vi "UHR-Fleezers Control (host) - 11.9.vi"() -> ()   [LabVIEW 2014] (continued)
                                n672 = Select(t=w978, s="Random Choice", f=w984) -> (s? t:f=w982:dbl)
                                n673 = Select(t="Yank to Trap D (MHz)", s="Yank to which?", f="Yank to SP") -> (s? t:f=w975:dbl[])
                                n674 = Index Array(array=w975, index=w982) -> (element=w985:dbl)
                                n675 = case shown="False" "Yank to which?" {
                                tunnel: w985 -> [w986 w1013]
                                frame False {
                                n676 = flat-sequence {
                                tunnel: w986 -> [w987]
                                frame #0 {
                                n677 = property on="Trap Pos FB SP" class="DigNum (strict)"("Val(Sgnl)"=w987) -> ()  [unwired: 2 in, 2 out]
                                }
                                frame #1 {
                                n678 = Wait (ms)(milliseconds to wait=u32 700) -> ()  [unwired: 1 out]
                                }
                                frame #2 {
                                n679 = local read "Action (%)"() -> (w992:dbl)
                                n680 = Absolute Value(x=w992) -> (abs(x)=w991:dbl)
                                n681 = Greater?(x=w991, y=70.0) -> (0:w989:bool)
                                n682 = property on="Remove Action Offset" class="Bool (strict)"("Val(Sgnl)"=w989) -> ()  [unwired: 2 in, 2 out]
                                }
                                frame #3 {
                                n683 = for {
                                N: 4 -> [_]
                                n684 = flat-sequence {
                                frame #0 {
                                n685 = Wait (ms)(milliseconds to wait=u32 500) -> ()  [unwired: 1 out]
                                }
                                frame #1 {
                                n686 = local read "Action (%)"() -> (w998:dbl)
                                n687 = Absolute Value(x=w998) -> (abs(x)=w997:dbl)
                                n688 = Greater?(x=w997, y=70.0) -> (0:w995:bool)
                                n689 = property on="Remove Action Offset" class="Bool (strict)"("Val(Sgnl)"=w995) -> ()  [unwired: 2 in, 2 out]
                                }
                                }
                                }
                                }
                                frame #4 {
                                n690 = local read "Shift confocal"() -> (w1002:bool)
                                n691 = local read "Mean"() -> (w1005:dbl)
                                n692 = Greater?(x=w1005, y=11.0) -> (0:w1001:bool)
                                n693 = Not(x=w1001) -> (.not. x?=w1000:bool)
                                n694 = And(x=w1000, y=w1002) -> (x .and. y?=w999:bool)
                                n695 = And(x=w1001, y=w1002) -> (x .and. y?=w1003:bool)
                                n696 = case shown="True" w1003 {
                                frame False {
                                }
                                frame True {
                                n697 = local read "Confocal X 2 (V)"() -> (w1008:dbl)
                                n698 = local read "Confocal Y 2 (V)"() -> (w1009:dbl)
                                n699 = property on="AO2" class="Slide (strict)"("Val(Sgnl)"=w1008) -> ()  [unwired: 2 in, 2 out]
                                n700 = property on="AO1" class="Slide (strict)"("Val(Sgnl)"=w1009) -> ()  [unwired: 2 in, 2 out]
                                }
                                }
                                n701 = case shown="True" w999 {
                                frame False {
                                }
                                frame True {
                                n702 = local read "Confocal X 1 (V)"() -> (w1006:dbl)
                                n703 = local read "Confocal Y 1 (V)"() -> (w1007:dbl)
                                n704 = property on="AO1" class="Slide (strict)"("Val(Sgnl)"=w1007) -> ()  [unwired: 2 in, 2 out]
                                n705 = property on="AO2" class="Slide (strict)"("Val(Sgnl)"=w1006) -> ()  [unwired: 2 in, 2 out]
                                }
                                }
                                }
                                frame #5 {
                                n706 = Wait (ms)(milliseconds to wait=u32 1500) -> ()  [unwired: 1 out]
                                }
                                frame #6 {
                                n707 = property on="Remove Offset" class="Bool (strict)"("Val(Sgnl)"=TRUE ("Value (Signaling)")) -> ()  [unwired: 2 in, 2 out]
                                n708 = property on="Rem fb disp offset" class="Bool (strict)"("Val(Sgnl)"=TRUE ("Value (Signaling)")) -> ()  [unwired: 2 in, 2 out]
                                }
                                }
                                }
                                frame True {
                                n709 = flat-sequence {
                                tunnel: w1013 -> [w1014]
                                frame #0 {
                                n710 = property on="Trap D (MHz)" class="DigNum (strict)"("Val(Sgnl)"=w1014) -> ()  [unwired: 2 in, 2 out]
                                }
                                frame #1 {
                                n711 = Wait (ms)(milliseconds to wait=u32 500) -> ()  [unwired: 1 out]
                                }
                                frame #2 {
                                n712 = local read "Shift confocal"() -> (w1018:bool)
                                n713 = local read "Mean"() -> (w1016:dbl)
                                n714 = Greater?(x=w1016, y=11.0) -> (0:w1019:bool)
                                n715 = Not(x=w1019) -> (.not. x?=w1020:bool)
                                n716 = And(x=w1020, y=w1018) -> (x .and. y?=w1022:bool)
                                n717 = And(x=w1019, y=w1018) -> (x .and. y?=w1021:bool)
                                n718 = case shown="True" w1021 {
                                frame False {
                                }
                                frame True {
                                n719 = local read "Confocal Y 2 (V)"() -> (w1026:dbl)
                                n720 = local read "Confocal X 2 (V)"() -> (w1025:dbl)
                                n721 = property on="AO1" class="Slide (strict)"("Val(Sgnl)"=w1026) -> ()  [unwired: 2 in, 2 out]
                                n722 = property on="AO2" class="Slide (strict)"("Val(Sgnl)"=w1025) -> ()  [unwired: 2 in, 2 out]
                                }
                                }
                                n723 = case shown="True" w1022 {
                                frame False {
                                }
                                frame True {
                                n724 = local read "Confocal X 1 (V)"() -> (w1023:dbl)
                                n725 = local read "Confocal Y 1 (V)"() -> (w1024:dbl)
                                n726 = property on="AO2" class="Slide (strict)"("Val(Sgnl)"=w1023) -> ()  [unwired: 2 in, 2 out]
                                n727 = property on="AO1" class="Slide (strict)"("Val(Sgnl)"=w1024) -> ()  [unwired: 2 in, 2 out]
                                }
                                }
                                }
                                }
                                }
                                }
                                }
                              }
                            }
                            frame "Raster" {
                              n728 = property on="Trap Raster Scan" class="Bool (strict)"("Val(Sgnl)"=TRUE ("Value (Signaling)")) -> ()  [unwired: 2 in, 2 out]
                            }
                          }
                          n729 = local read "Time (s)"() -> (w959:dbl)
                          "Fl. High" <- TRUE ("Yanking")
                        }
                        frame #1 {
                          n730 = local read "Auto F Reset"() -> (w1028:bool)
                          n731 = case shown="True" w1028 {
                            tunnel: w1033 -> [_ w1037]
                            tunnel: w1032 -> [_ w1036]
                            tunnel: w1031 -> [_ w1035]
                            tunnel: w1029 -> [_ w1034]
                            frame False {
                            }
                            frame True {
                              n732 = node-c288() -> (w1039:T21)  [unwired: 4 out]
                              n733 = timed-loop {
                                timing: w1039 -> [_]
                                timing-out: [_] -> w1038
                                tunnel: w1037 -> [w1057]
                                tunnel: w1036 -> [w1056]
                                tunnel: w1035 -> [w1055]
                                tunnel: w1034 -> [w1054]
                                stop <- w1040 stop-if-true
                                n734 = node-c288() -> ()  [unwired: 2 out]
                                n735 = local read "Fl. D Thresh. (kHz)"() -> (w1048:dbl)
                                n736 = local read "Fl. Triggered..."() -> (w1053:bool)
                                n737 = local read "Delta Fl. 1"() -> (w1044:dbl)
                                n738 = local read "Delta Fl. 2"() -> (w1042:dbl)
                                n739 = local read "Stop All"() -> (w1051:bool)
                                n740 = local read "APD to Watch"() -> (w1043:bool)
                                n741 = Select(t=w1044, s=w1043, f=w1042) -> (s? t:f=w1041:dbl)
                                n742 = Not(x=w1053) -> (.not. x?=w1052:bool)
                                n743 = Multiply(x=w1048, y=1000.0) -> (x*y=w1047:dbl)
                                n744 = Negate(x=w1047) -> (-x=w1046:dbl)
                                n745 = Less?(x=w1041, y=w1046) -> (x < y?=w1050:bool)
                                n746 = Compound Arithmetic op=OR(w1050, w1051, w1052, "Reset Force") -> (w1040:bool)
                                n747 = case shown="True" w1040 {
                                tunnel: w1057 -> [_ w1072]
                                tunnel: w1056 -> [_ w1071]
                                tunnel: w1055 -> [_ w1061]
                                tunnel: w1054 -> [_ w1063]
                                frame False {
                                }
                                frame True {
                                n748 = local read "Time (s)"() -> (w1062:dbl)
                                n749 = case shown="\"Yank\"" w1071 {
                                tunnel: w1072 -> [_ w1075]
                                tunnel: w1063 -> [_ w1073]
                                frame "Image", Default {
                                }
                                frame "Yank" {
                                n750 = flat-sequence {
                                tunnel: [w1081] -> w1076
                                tunnel: w1075 -> [w1081]
                                tunnel: [w1077] -> w1074
                                tunnel: w1073 -> [w1077]
                                tunnel: w1076 -> [w1084]
                                tunnel: w1074 -> [w1082]
                                frame #0 {
                                n751 = local read "Yank Delay (s)"() -> (w1080:dbl)
                                n752 = Multiply(x=w1080, y=1000.0) -> (x*y=w1078:dbl)
                                n753 = Wait (ms)(milliseconds to wait=w1078) -> ()  [unwired: 1 out]
                                }
                                frame #1 {
                                n754 = local read "Yank to which?"() -> (w1083:bool)
                                n755 = case shown="False" w1083 {
                                tunnel: w1084 -> [_ w1112]
                                tunnel: w1082 -> [w1085 _]
                                frame False {
                                n756 = flat-sequence {
                                tunnel: w1085 -> [w1086]
                                frame #0 {
                                n757 = property on="Trap Pos FB SP" class="DigNum (strict)"("Val(Sgnl)"=w1086) -> ()  [unwired: 2 in, 2 out]
                                }
                                frame #1 {
                                n758 = Wait (ms)(milliseconds to wait=u32 700) -> ()  [unwired: 1 out]
                                }
                                frame #2 {
                                n759 = local read "Action (%)"() -> (w1091:dbl)
                                n760 = Absolute Value(x=w1091) -> (abs(x)=w1090:dbl)
                                n761 = Greater?(x=w1090, y=70.0) -> (0:w1088:bool)
                                n762 = property on="Remove Action Offset" class="Bool (strict)"("Val(Sgnl)"=w1088) -> ()  [unwired: 2 in, 2 out]
                                }
                                frame #3 {
                                n763 = for {
                                N: 4 -> [_]
                                n764 = flat-sequence {
                                frame #0 {
                                n765 = Wait (ms)(milliseconds to wait=u32 500) -> ()  [unwired: 1 out]
                                }
                                frame #1 {
                                n766 = local read "Action (%)"() -> (w1097:dbl)
                                n767 = Absolute Value(x=w1097) -> (abs(x)=w1096:dbl)
                                n768 = Greater?(x=w1096, y=70.0) -> (0:w1094:bool)
                                n769 = property on="Remove Action Offset" class="Bool (strict)"("Val(Sgnl)"=w1094) -> ()  [unwired: 2 in, 2 out]
                                }
                                }
                                }
                                }
                                frame #4 {
                                n770 = local read "Shift confocal"() -> (w1102:bool)
                                n771 = local read "Mean"() -> (w1104:dbl)
                                n772 = Greater?(x=w1104, y=11.0) -> (0:w1101:bool)
                                n773 = Not(x=w1101) -> (.not. x?=w1100:bool)
                                n774 = And(x=w1101, y=w1102) -> (x .and. y?=w1099:bool)
                                n775 = And(x=w1100, y=w1102) -> (x .and. y?=w1098:bool)
                                n776 = case shown="True" w1099 {
                                frame False {
                                }
                                frame True {
                                n777 = local read "Confocal Y 2 (V)"() -> (w1108:dbl)
                                n778 = local read "Confocal X 2 (V)"() -> (w1107:dbl)
                                n779 = property on="AO2" class="Slide (strict)"("Val(Sgnl)"=w1107) -> ()  [unwired: 2 in, 2 out]
                                n780 = property on="AO1" class="Slide (strict)"("Val(Sgnl)"=w1108) -> ()  [unwired: 2 in, 2 out]
                                }
                                }
                                n781 = case shown="True" w1098 {
                                frame False {
                                }
                                frame True {
                                n782 = local read "Confocal X 1 (V)"() -> (w1105:dbl)
                                n783 = local read "Confocal Y 1 (V)"() -> (w1106:dbl)
                                n784 = property on="AO1" class="Slide (strict)"("Val(Sgnl)"=w1106) -> ()  [unwired: 2 in, 2 out]
                                n785 = property on="AO2" class="Slide (strict)"("Val(Sgnl)"=w1105) -> ()  [unwired: 2 in, 2 out]
                                }
                                }
                                }
                                frame #5 {
                                n786 = Wait (ms)(milliseconds to wait=u32 1500) -> ()  [unwired: 1 out]
                                }
                                frame #6 {
                                n787 = property on="Rem fb disp offset" class="Bool (strict)"("Val(Sgnl)"=TRUE ("Value (Signaling)")) -> ()  [unwired: 2 in, 2 out]
                                n788 = property on="Remove Offset" class="Bool (strict)"("Val(Sgnl)"=TRUE ("Value (Signaling)")) -> ()  [unwired: 2 in, 2 out]
                                }
                                }
                                }
                                frame True {
                                n789 = flat-sequence {
                                tunnel: w1112 -> [w1113]
                                frame #0 {
                                n790 = property on="Trap D (MHz)" class="DigNum (strict)"("Val(Sgnl)"=w1113) -> ()  [unwired: 2 in, 2 out]
                                }
                                frame #1 {
                                n791 = Wait (ms)(milliseconds to wait=u32 500) -> ()  [unwired: 1 out]
                                }
                                frame #2 {
                                n792 = local read "Shift confocal"() -> (w1119:bool)
                                n793 = local read "Mean"() -> (w1121:dbl)
                                n794 = Greater?(x=w1121, y=11.0) -> (0:w1118:bool)
                                n795 = Not(x=w1118) -> (.not. x?=w1117:bool)
                                n796 = And(x=w1118, y=w1119) -> (x .and. y?=w1116:bool)
                                n797 = And(x=w1117, y=w1119) -> (x .and. y?=w1115:bool)
                                n798 = case shown="True" w1116 {
                                frame False {
                                }
                                frame True {
                                n799 = local read "Confocal Y 2 (V)"() -> (w1125:dbl)
                                n800 = local read "Confocal X 2 (V)"() -> (w1124:dbl)
                                n801 = property on="AO2" class="Slide (strict)"("Val(Sgnl)"=w1124) -> ()  [unwired: 2 in, 2 out]
                                n802 = property on="AO1" class="Slide (strict)"("Val(Sgnl)"=w1125) -> ()  [unwired: 2 in, 2 out]
                                }
                                }
                                n803 = case shown="True" w1115 {
                                frame False {
                                }
                                frame True {
                                n804 = local read "Confocal Y 1 (V)"() -> (w1123:dbl)
                                n805 = local read "Confocal X 1 (V)"() -> (w1122:dbl)
                                n806 = property on="AO2" class="Slide (strict)"("Val(Sgnl)"=w1122) -> ()  [unwired: 2 in, 2 out]
                                n807 = property on="AO1" class="Slide (strict)"("Val(Sgnl)"=w1123) -> ()  [unwired: 2 in, 2 out]
                                }
                                }
                                }
                                }
                                }
                                }
                                }
                                }
                                }
                                }
                                n808 = local read "Messages"() -> (w1070:string)
                                n809 = Subtract(x=w1062, y=w1061) -> (x-y=w1068:dbl)
                                "Duration (s)" <- w1068
                                n810 = Number To Decimal String(number=w1068, width (-)=i16 0) -> (decimal integer string=w1066:string)
                                n811 = Concatenate Strings(w1066, " s fluorescence event." ("string")) -> (w1064:string)
                                n812 = call "Update messages.vi"("Message to add"=w1064, "Old message string"=w1070) -> ("New message string"=w1069:string)
                                n813 = local write "Reset Force"(FALSE ("Reset Force")) -> ()
                                n814 = local write "Waiting"(TRUE ("Waiting")) -> ()
                                n815 = local write "Messages"(w1069) -> ()
                                n816 = local write "Fl. High"(FALSE ("Fl. High")) -> ()
                                n817 = call <vilib>:"Beep.vi"() -> ()  [unwired: 3 in, 9 out]
                                }
                                }
                                n818 = node-c288() -> ()  [unwired: 2 out]
                              }
                              n819 = node-c288(w1038) -> ()  [unwired: 1 out]
                            }
                          }
                        }
                      }
                      n820 = local read "Trap Pos FB SP"() -> (w946:fxp<+/-,16,1>)
                      n821 = local read "Trap D (MHz)"() -> (w951:dbl)
                    }
                  }
                }
                frame #1 {
                  n822 = local read "Stop All"() -> (w1135:bool)
                  n823 = local read "Fl. Triggered..."() -> (w1133:bool)
                  n824 = Not(x=w1133) -> (.not. x?=w1134:bool)
                  n825 = Or(x=w1134, y=w1135) -> (x .or. y?=w1132:bool)
                }
              }
              n826 = case shown="True" w721 {
                frame False {
                }
                frame True {
                  n827 = local read "Confocal Y 1 (V)"() -> (w731:dbl)
                  n828 = local read "Confocal X 1 (V)"() -> (w730:dbl)
                  n829 = property on="AO2" class="Slide (strict)"("Val(Sgnl)"=w730) -> ()  [unwired: 2 in, 2 out]
                  n830 = property on="AO1" class="Slide (strict)"("Val(Sgnl)"=w731) -> ()  [unwired: 2 in, 2 out]
                }
              }
              n831 = case shown="True" w721 {
                frame False {
                }
                frame True {
                  w729 = FALSE ("Fl. High")
                  n832 = local write "Waiting"(w729) -> ()
                  n833 = local write "Fl. High"(w729) -> ()
                }
              }
              n834 = node-c288() -> ()  [unwired: 2 out]
            }
            n835 = node-c288(w719) -> ()  [unwired: 1 out]
          }
        }
      }
      event "Stop All": Value Change {
        n836 = event-data() -> ()  [unwired: 7 out]
        n837 = local read "Stop All"() -> (w1140:bool)
      }
    }
    n838 = node-c288() -> ()  [unwired: 2 out]
  }
  n839 = property on="Saved trap pos" class="WFGraph (strict)"("Visible"=TRUE) -> ()  [unwired: 2 in, 2 out]
  n840 = property on="Trap Delta Graph" class="WFGraph (strict)"("Visible"=FALSE) -> ()  [unwired: 2 in, 2 out]
  n841 = local write "Trap pos"(TRUE ("Trap pos")) -> ()
  n842 = node-c288(2 ("Processor")) -> (w110:T21)  [unwired: 3 out]
  n843 = timed-loop "Control parameters (event loop)" {
    tunnel: w20 -> [w1149]
    shift-right: [w1148] -> _
    shift-left: errorcluster {"status"=FALSE, "code"=0, "source"=""} ("error out") -> [w1147]
    tunnel: [w1146] -> _
    timing: w110 -> [_]
    timing-out: [_] -> w109
    tunnel: w83 -> [w1145]
    tunnel: w24 -> [w1144]
    tunnel: w23 -> [w1143]
    tunnel: w22 -> [w1142]
    tunnel: w21 -> [w1141]
    stop <- w1146 stop-if-true
    n844 = node-c288() -> ()  [unwired: 2 out]
    n845 = event shown="[77] \"Save user params\": Value Change" {
      selector: _ -> [_ _ _ _ _ _ _ _ _ _ _ _ _ _ _ _ _ _ _ _ _ _ _ _ _ _ _ _ _ _ _ _ _ _ _ _ _ _ _ _ _ _ _ _ _ _ _ _ _ _ _ _ _ _ _ _ _ _ _ _ _ _ _ _ _ _ _ _ _ _ _ _ _ _ _ _ _ _ _ _]
      dyn-events: _ -> [_ _ _ _ _ _ _ _ _ _ _ _ _ _ _ _ _ _ _ _ _ _ _ _ _ _ _ _ _ _ _ _ _ _ _ _ _ _ _ _ _ _ _ _ _ _ _ _ _ _ _ _ _ _ _ _ _ _ _ _ _ _ _ _ _ _ _ _ _ _ _ _ _ _ _ _ _ _ _ _]
      timeout: _ -> [_ _ _ _ _ _ _ _ _ _ _ _ _ _ _ _ _ _ _ _ _ _ _ _ _ _ _ _ _ _ _ _ _ _ _ _ _ _ _ _ _ _ _ _ _ _ _ _ _ _ _ _ _ _ _ _ _ _ _ _ _ _ _ _ _ _ _ _ _ _ _ _ _ _ _ _ _ _ _ _]
      tunnel: w1149 -> [w1187 _ _ _ w1225 _ w1247 _ _ _ _ w1313 _ _ w1356 w1362 w1367 w1373 w1409 w1427 w1434 _ w1446 w1450 w1461 w1472 w1483 w1494 w1505 w1516 w1543 w1637 w1644 w1682 _ _ w1742 w1746 w1757 w1761 w1765 _ w1773 _ _ _ _ _ _ _ _ _ _ _ _ _ _ _ _ _ w2154 _ w2171 _ w2178 w2196 _ w2203 w2211 w2226 w2237 w2243 _ w2252 _ w2271 _ _ _ w2346]
      tunnel: [w1186 _ _ _ w1215 _ w1246 _ _ w1278 _ w1292 _ _ w1355 w1358 w1364 w1370 w1408 w1425 w1433 _ w1444 _ w1455 w1466 w1477 w1488 w1499 w1510 w1541 w1635 w1642 w1680 _ _ w1740 w1744 w1747 w1759 w1763 _ w1771 _ _ _ _ _ _ _ _ _ _ _ _ _ _ _ _ _ w2152 _ _ _ _ w2193 _ _ _ _ _ _ _ _ _ _ _ _ _ w2344] -> w1148
      tunnel: w1147 -> [w1185 _ _ _ w1224 _ w1245 _ _ w1278 _ w1312 _ _ w1354 w1357 w1363 w1369 w1407 w1426 w1432 _ w1445 w1449 w1460 w1471 w1482 w1493 w1504 w1515 w1542 w1636 w1643 w1681 _ _ w1741 w1745 w1756 w1760 w1764 _ w1772 _ _ _ _ _ _ _ _ _ _ _ _ _ _ _ _ _ w2153 _ w2170 _ w2177 w2195 _ w2202 w2210 w2225 w2236 w2242 _ w2251 _ w2270 _ _ _ w2345]
      tunnel: [_ _ _ _ _ _ _ _ _ w1277 _ _ _ _ _ _ _ _ _ _ _ _ _ _ _ _ _ _ _ _ _ _ _ _ _ _ _ _ _ _ _ _ _ _ _ _ _ _ _ _ _ _ _ _ _ _ _ _ _ _ _ _ _ _ _ _ _ _ _ _ _ _ _ _ _ _ _ _ _ _] -> w1146
      tunnel: [_ _ _ _ _ _ _ "Round T1 X" _ _ _ _ _ _ _ _ _ _ _ _ _ _ _ _ _ _ _ _ _ _ _ _ _ _ _ _ _ _ _ _ _ _ _ _ _ _ _ _ _ _ _ _ _ _ _ _ _ _ _ _ _ _ _ _ _ _ _ _ _ _ _ _ _ _ _ _ _ _ _ _] -> _
      tunnel: [_ _ _ "Adjust Scale\nto Mean" _ _ _ _ _ _ _ _ _ _ _ _ _ _ _ _ _ _ "Test ttrig" _ _ _ _ _ _ _ _ _ _ _ _ _ _ _ _ _ _ _ _ _ _ _ _ _ _ _ "Flush Sample" "Flush Pump 3" "Flush Pump 1" "Clear Volume" _ _ _ _ _ _ _ _ _ _ _ _ _ _ _ _ _ _ _ _ _ _ _ _ _ _] -> _
      tunnel: [_ _ _ _ _ _ _ _ "Round T2 X" _ "Delayed Interlace Start" _ _ _ _ _ _ _ _ _ _ _ _ _ _ _ _ _ _ _ _ _ _ _ _ _ _ _ _ _ _ _ _ _ _ _ _ _ _ _ _ _ _ _ _ _ _ _ _ _ _ _ _ _ _ _ _ _ _ _ _ _ _ _ _ _ _ _ _ _] -> _
      tunnel: w1145 -> [_ _ _ _ _ _ _ _ _ _ _ _ _ _ _ _ _ _ _ _ _ _ _ _ _ _ _ _ _ _ _ _ _ _ _ _ _ _ _ _ _ _ _ _ _ _ w1931 w1949 w1956 w1961 w1967 _ _ w2066 _ _ _ _ _ _ _ _ _ _ _ _ _ _ _ _ _ _ _ _ _ _ _ _ _ _]
      tunnel: w1144 -> [_ _ _ _ _ _ _ _ _ _ _ _ _ _ _ _ _ _ _ _ _ _ _ _ _ _ _ _ _ _ _ _ _ _ _ _ _ _ _ _ _ _ _ _ w1847 _ _ _ _ _ _ w1997 _ _ w2073 _ w2082 _ w2096 _ _ _ _ _ _ _ _ _ _ _ _ _ _ _ _ _ _ _ _ _]
      tunnel: w1143 -> [_ _ _ _ _ _ _ _ _ _ _ _ _ _ _ _ _ _ _ _ _ _ _ _ _ _ _ _ _ _ _ _ _ _ _ _ _ _ _ _ _ _ _ _ _ _ _ _ _ _ _ _ _ _ _ _ _ _ _ _ _ _ _ _ _ _ _ _ _ _ _ _ _ _ _ _ _ _ _ _]
      tunnel: w1142 -> [_ _ _ _ _ _ _ _ _ _ _ _ _ _ _ _ _ _ _ _ _ _ _ _ _ _ _ _ _ _ _ _ _ _ _ _ _ _ _ _ _ _ _ w1784 _ _ _ _ _ _ _ _ w2027 _ _ w2078 _ w2089 _ w2121 _ _ _ _ _ _ _ _ _ _ _ _ _ _ _ _ _ _ _ _]
      tunnel: w1141 -> [_ _ _ _ _ _ _ _ _ _ _ _ _ _ _ _ _ _ _ _ _ _ _ _ _ _ _ _ _ _ _ _ _ _ _ _ _ _ _ _ _ _ _ _ _ _ _ _ _ _ _ _ _ _ _ _ _ _ _ _ _ _ _ _ _ _ _ _ _ _ _ _ _ _ _ _ _ _ _ _]
      event "AI Count (ticks)", "Sets to FIFO (Traps)", "Save ave N", "FPGA Ave.", "# Samples/channel", "N sets to save": Value Change {
        # "So that if 'Save ave N' is updated, the AOD scanning code updates too."
        n846 = event-data() -> ()  [unwired: 6 out]
        n847 = local read "AI Count (ticks)"() -> (w1167:u32)
        n848 = Boolean To (0,1)(Boolean="Sets to FIFO (Traps)") -> (0, 1=w1177:cluster{"Set 1":i16, "Set 2":i16, "Set 3":i16})
        n849 = Cluster To Array(cluster=w1177) -> (array=w1176:i16[])
        n850 = xnode "Read/Write Control"("FPGA VI Reference In"=w1187, "error in"=w1185, "ai count"=w1167, "AI1 Sets to FIFO"="Sets to FIFO (Traps)", "N of AI1 Int Acq Sets"="N Acq Sets (Traps + Fl.)") -> ("error out"=w1186:errorcluster)  [unwired: 1 out]
        n851 = To Unsigned Long Integer(number=w1176) -> (unsigned 32bit integer=w1156:u32[])
        n852 = local read "Scan steps (AOD)"() -> (w1178:u64)
        n853 = Multiply(x=w1167, y="N Acq Sets (Traps + Fl.)") -> (x*y=w1165:u32)
        n854 = Divide(x=40000000.0, y=w1167) -> (x/y=w1159:dbl)
        "AI rate (Hz)" <- w1159
        "Ave. Rate (Hz)" <- w1159
        n855 = Add Array Elements(numeric array=w1156) -> (sum=w1168:u32)
        "Trap Sets" <- w1168
        n856 = Reciprocal(x=w1159) -> (1/x=→"Ave. Period (s)":dbl)
        n857 = property on="Scan steps (AOD)" class="DigNum (strict)"("Val(Sgnl)"=w1178) -> ()  [unwired: 2 in, 2 out]
        n858 = Divide(x=w1159, y="N Acq Sets (Traps + Fl.)") -> (x/y=w1182:dbl)
        "Data Rate (Hz)" <- w1182
        n859 = Reciprocal(x=w1182) -> (1/x=→"Data Period (s)":dbl)
        n860 = local read "Save ave N"() -> (w1181:dbl)
        n861 = Divide(x=w1182, y=w1181) -> (x/y=w1180:dbl)
        "Save Data Rate (Hz)" <- w1180
        n862 = Reciprocal(x=w1180) -> (1/x=→"Save Data Period (s)":dbl)
        n863 = Multiply(x=w1165, y="# Samples/trap") -> (x*y=w1163:u32)
        "Counts/DMA" <- w1163
        n864 = property on="Trap Disp. Downsample" class="DigNum (strict)"("Maximum"="# Samples/trap") -> ()  [unwired: 2 in, 2 out]
        n865 = Multiply(x=w1168, y="# Samples/trap") -> (x*y=w1157:u32)
        "# Samples/channel" <- w1157
        n866 = Multiply(x=w1157, y=u32 8) -> (x*y=→"Trap AI Elements/DMA read":u32)
        n867 = local read "APD Int. Count"() -> (w1164:u32)
        n868 = Multiply(x=w1157, y=u32 3) -> (x*y=→"Trap Pos Elements/DMA read":u32)
        n869 = Divide(x=w1163, y=w1164) -> (x/y=w1154:dbl)
        "APD Samples/FIFO Acq." <- w1154
        n870 = Divide(x=w1163, y=40000000.0) -> (x/y=w1161:dbl)
        "DMA Update Period (s)" <- w1161
        n871 = Multiply(x=2.0, y=w1154) -> (x*y=→"APD Elements/DMA read":dbl)
        n872 = property on="APD Disp. Downsample" class="DigNum (strict)"("Maximum"=w1154) -> ()  [unwired: 2 in, 2 out]
        n873 = local read "N sets to save"() -> (w1174:u32)
        n874 = Multiply(x=w1161, y=w1174) -> (x*y=→"Total Time (s)":dbl)
        "FPGA Averaging" <- FALSE ("FPGA Averaging")
      }
      event "Remove Offset": Value Change {
        n875 = event-data() -> ()  [unwired: 7 out]
        n876 = local write "Remove Offset"(FALSE ("Remove Offset")) -> ()
        n877 = local read "Bead Mean (nm)"() -> (w1189:dbl)
        n878 = local read "Offset (nm)"() -> (w1190:dbl)
        n879 = Add(x=w1189, y=w1190) -> (x+y=w1188:dbl)
        n880 = local write "Offset (nm)"(w1188) -> ()
        n881 = disable-structure shown="Disabled" {
          frame Disabled {
            n882 = local read "Bead Mean (nm)"() -> (w1195:dbl)
            n883 = Add(y=w1195) -> (x=w1194:dbl, x+y=w1193:dbl)
            n884 = Subtract(x=w1195, y=w1194) -> (x-y=w1192:dbl)
            n885 = property on="Bead Separation" class="WFChart (strict)"("YScale.Minimum"=w1192) -> ()  [unwired: 2 in, 2 out]
            n886 = property on="Bead Separation" class="WFChart (strict)"("YScale.Maximum"=w1193) -> ()  [unwired: 2 in, 2 out]
          }
          frame Enabled {
          }
        }
      }
      event "Detector Type": Value Change {
        n887 = event-data() -> ()  [unwired: 7 out]
        n888 = local read "AI labels"() -> (w1196:string[])
        n889 = property on="High Res. Display" class="Ring (strict)"("Strings []"=w1196) -> ()  [unwired: 2 in, 2 out]
        n890 = Build Array (concatenate)(w1196, "none") -> (w1197:string[])
        n891 = property on="FFT 1 Choice 1" class="Ring (strict)"("Strings []"=w1197) -> ()  [unwired: 2 in, 2 out]
        n892 = property on="FFT 1 Choice 2" class="Ring (strict)"("Strings []"=w1197) -> ()  [unwired: 2 in, 2 out]
        n893 = property on="FFT 2 Choice 1" class="Ring (strict)"("Strings []"=w1197) -> ()  [unwired: 2 in, 2 out]
        n894 = property on="FFT 2 Choice 2" class="Ring (strict)"("Strings []"=w1197) -> ()  [unwired: 2 in, 2 out]
        n895 = Bundle("APD 1", "APD 2") -> (w1200:cluster{string, string})  [unwired: 1 out]
        n896 = Cluster To Array(cluster=w1200) -> (array=w1198:string[])
        n897 = Build Array (concatenate)(w1198, w1197) -> (w1202:string[])
        n898 = Array Size(array=w1202) -> (size(s)=w1203:i32)
        n899 = property on="Signals to Plot" class="LstBox (strict)"("Item Names"=w1202) -> ()  [unwired: 2 in, 2 out]
        n900 = property on="Signals to Plot" class="LstBox (strict)"("Number of Rows"=w1203) -> ()  [unwired: 2 in, 2 out]
        n901 = property on="All Signals" class="WFChart (strict)"("LegNumRows"=w1203) -> ()  [unwired: 2 in, 2 out]
      }
      event "Adjust Scale\nto Mean": Value Change {
        n902 = event-data() -> ()  [unwired: 7 out]
        n903 = local read "APD 1 Rate (Hz)"() -> (w1212:dbl)
        n904 = Multiply(x=1000.0, y="Above (kHz)") -> (x*y=w1210:dbl)
        n905 = Multiply(x=1000.0, y="Below (kHz)") -> (x*y=w1208:dbl)
        n906 = Add(x=w1210, y=w1212) -> (x+y=w1205:dbl)
        n907 = Subtract(x=w1212, y=w1208) -> (x-y=w1206:dbl)
        n908 = property on="APD Chart" class="WFChart (strict)"("YScale.Minimum"=w1206) -> ()  [unwired: 2 in, 2 out]
        n909 = property on="APD Chart" class="WFChart (strict)"("YScale.Maximum"=w1205) -> ()  [unwired: 2 in, 2 out]
      }
      event "Phase adj. (AI1)", "+ phase (AI1)", "- phase (AI1)": Value Change {
        n910 = event-data() -> ()  [unwired: 7 out]
        n911 = Negate(x="Phase adj. (AI1)") -> (-x=w1222:i16)
        n912 = Select(t=w1222, s="- phase (AI1)", f="Phase adj. (AI1)") -> (s? t:f=w1221:i16)
        n913 = xnode "Read/Write Control"("FPGA VI Reference In"=w1225, "error in"=w1224, "Phase count adjustment"=w1221) -> ("FPGA VI Reference Out"=w1220:T19, "error out"=w1219:errorcluster)
        n914 = Or(x="- phase (AI1)", y="+ phase (AI1)") -> (x .or. y?=w1216:bool)
        n915 = xnode "Read/Write Control"("FPGA VI Reference In"=w1220, "error in"=w1219, "+ phase"=w1216) -> ("error out"=w1215:errorcluster)  [unwired: 1 out]
      }
      event "Signals to Plot": Double Click {
        w1228 = u32 9868950 ("Color Box")
        n916 = event-data() -> ("Row"=w1230:i32)  [unwired: 9 out]
        n917 = property on="All Signals" class="WFChart (strict)"("Active Plot"=w1230) -> (error out=w1241:errorcluster)  [unwired: 2 in, 1 out]
        n918 = property on="All Signals" class="WFChart (strict)" props=["Plot", "Visible?", "Plot", "Plot Color"](error in=w1241) -> (error out=w1240:errorcluster, "Plot.Visible?"=w1239:bool)  [unwired: 1 in, 2 out]
        n919 = Select(t=FALSE ("Plot.Visible"), s=w1239, f=TRUE ("Plot.Visible")) -> (s? t:f=w1234:bool)
        n920 = property on="All Signals" class="WFChart (strict)"(error in=w1240, "Plot.Visible?"=w1234) -> (error out=w1236:errorcluster)  [unwired: 1 in, 1 out]
        n921 = property on="All Signals" class="WFChart (strict)"(error in=w1236) -> (error out=w1231:errorcluster, "Plot.Plot Color"=w1235:u32)  [unwired: 1 in, 1 out]
        n922 = property on="Signals to Plot" class="LstBox (strict)"(error in=w1231, "Active Row"=w1230) -> (error out=w1229:errorcluster)  [unwired: 1 in, 1 out]
        n923 = Select(t=w1235, s=w1234, f=u32 0) -> (s? t:f=w1232:u32)
        n924 = property on="Signals to Plot" class="LstBox (strict)"(error in=w1229, "CellFontColor"=w1232, "SelColor"=w1228, "CellBG"=w1228, "CellFontSize"=u32 20 ("Active Row:Cell Font:Size"), "CellFontBold"=TRUE ("Active Row:Cell Font:Bold")) -> ()  [unwired: 1 in, 2 out]
      }
      event "BD 1 Frequency 1 (MHz)", "BD 1 Frequency 2 (MHz)", "BD 1 Frequency 3 (MHz)", "BD 2 Frequency 1 (MHz)", "BD 2 Frequency 2 (MHz)", "BD 2 Frequency 3 (MHz)", "Trap D (MHz)": Value Change {
        n925 = event-data() -> ("CtlRef"=w1244:refnum<vi>)  [unwired: 6 out]
        n926 = control-ref of="Trap D (MHz)"() -> (w1243:refnum<vi>)
        n927 = Equal?(x=w1243, y=w1244) -> (x = y?=w1242:bool)
        n928 = case shown="False" "Oscillate Set 1" {
          tunnel: w1247 -> [w1267 _]
          tunnel: [w1266 w1270] -> w1246
          tunnel: w1245 -> [w1265 w1270]
          tunnel: w1242 -> [w1250 _]
          frame False {
            n929 = local read "BD 1 Frequency 2 (MHz)"() -> (w1254:dbl)
            n930 = local read "BD 1 Frequency 1 (MHz)"() -> (w1252:dbl)
            n931 = Subtract(x=w1254, y="Trap D (MHz)") -> (x-y=w1251:dbl)
            n932 = Select(t=w1251, s=w1250, f=w1252) -> (s? t:f=w1249:dbl)
            n933 = local read "Y RF Frequency Limits (MHz)"() -> (w1255:T16)
            n934 = local read "X RF Frequency Limits (MHz)"() -> (w1256:T16)
            n935 = local read "BD 1 Frequency 3 (MHz)"() -> (w1268:dbl)
            n936 = local write "BD 1 Frequency 1 (MHz)"(w1249) -> ()
            n937 = local read "BD 2 Frequency 1 (MHz)"() -> (w1259:dbl)
            n938 = local read "BD 2 Frequency 2 (MHz)"() -> (w1258:dbl)
            n939 = local read "BD 2 Frequency 3 (MHz)"() -> (w1269:dbl)
            n940 = call "set RF board frequency - interlace.vi"("Board 2 Frequency Limits"=w1255, "Board 1 Frequency Limits"=w1256, "error in"=w1265, "FPGA VI Reference In"=w1267, "Board 2 Frequency 3 (MHz)"=w1269, "Board 1 Frequency 3 (MHz)"=w1268, "Board 2 Frequency 2 (MHz)"=w1258, "Board 2 Frequency 1 (MHz)"=w1259, "Board 1 Frequency 2 (MHz)"=w1254, "Board 1 Frequency 1  (MHz)"=w1249) -> ("error out"=w1266:errorcluster)  [unwired: 1 out]
            n941 = Subtract(x=w1259, y=w1258) -> (x-y=w1263:dbl)
            n942 = Subtract(x=w1249, y=w1254) -> (x-y=w1264:dbl)
            n943 = Square(x=w1263) -> (x^2=w1261:dbl)
            n944 = Square(x=w1264) -> (x^2=w1262:dbl)
            n945 = Add(x=w1262, y=w1261) -> (x+y=w1260:dbl)
            n946 = Square Root(x=w1260) -> (sqrt(x)=w1257:dbl)
            n947 = local write "Trap D (MHz)"(w1257) -> ()
            n948 = property on="Initial D (MHz)" class="DigNum (strict)"("Val(Sgnl)"=w1257) -> ()  [unwired: 2 in, 2 out]
          }
          frame True {
          }
        }
      }
      event "Round T1 X": Value Change {
        n949 = event-data() -> ()  [unwired: 7 out]
        n950 = local read "BD 1 Frequency 1 (MHz)"() -> (w1273:dbl)
        n951 = Round To Nearest(number=w1273) -> (nearest integer value=w1272:dbl)
        n952 = property on="BD 1 Frequency 1 (MHz)" class="DigNum (strict)"("Val(Sgnl)"=w1272) -> ()  [unwired: 2 in, 2 out]
      }
      event "Round T2 X": Value Change {
        n953 = event-data() -> ()  [unwired: 7 out]
        n954 = local read "BD 1 Frequency 2 (MHz)"() -> (w1275:dbl)
        n955 = Round To Nearest(number=w1275) -> (nearest integer value=w1274:dbl)
        n956 = property on="BD 1 Frequency 2 (MHz)" class="DigNum (strict)"("Val(Sgnl)"=w1274) -> ()  [unwired: 2 in, 2 out]
      }
      event "Stop All": Value Change {
        n957 = event-data() -> ()  [unwired: 7 out]
        n958 = local read "Stop All"() -> (w1277:bool)
      }
      event "Delayed Interlace Start": Value Change {
        n959 = event-data() -> ()  [unwired: 7 out]
        n960 = flat-sequence {
          frame #0 {
            n961 = Multiply(x="Delay to Interlace (s)", y=1000.0) -> (x*y=w1280:dbl)
            n962 = Wait (ms)(milliseconds to wait=w1280) -> ()  [unwired: 1 out]
          }
          frame #1 {
            n963 = property on="Green laser mode" class="RadioBtnsControl (strict)"("Val(Sgnl)"=enum32{"Laser ON", "Laser OFF", "Interlace"}."Interlace" ("Value (Signaling)")) -> ()  [unwired: 2 in, 2 out]
          }
        }
      }
      event "BD 1 Amplitude 1 (%)", "BD 1 Amplitude 2 (%)", "BD 1 Amplitude 3 (%)", "BD 2 Amplitude 1 (%)", "BD 2 Amplitude 2 (%)", "BD 2 Amplitude 3 (%)", "Trap 1 ON", "Trap 2 ON", "Trap 3 ON", "Feedback On/Off", "All FB On/Off": Value Change {
        w1304 = i16 1 ("f")
        n964 = event-data() -> ()  [unwired: 7 out]
        n965 = local write "Trap 1 (ON/OFF)"("Trap 1 ON") -> ()
        n966 = local write "Trap 2 (ON/OFF)"("Trap 2 ON") -> ()
        n967 = Boolean To (0,1)(Boolean="Trap 3 ON") -> (0, 1=w1305:i16)
        n968 = Boolean To (0,1)(Boolean="Trap 1 ON") -> (0, 1=w1306:i16)
        n969 = Boolean To (0,1)(Boolean="Trap 2 ON") -> (0, 1=w1307:i16)
        n970 = Select(t=w1307, s="Trap ON/OFF X or Y Amp?", f=w1304) -> (s? t:f=w1302:i16)
        n971 = Select(t=w1306, s="Trap ON/OFF X or Y Amp?", f=w1304) -> (s? t:f=w1303:i16)
        n972 = Select(t=w1305, s="Trap ON/OFF X or Y Amp?", f=w1304) -> (s? t:f=w1301:i16)
        n973 = Select(t=w1304, s="Trap ON/OFF X or Y Amp?", f=w1307) -> (s? t:f=w1299:i16)
        n974 = Select(t=w1304, s="Trap ON/OFF X or Y Amp?", f=w1306) -> (s? t:f=w1300:i16)
        n975 = Select(t=w1304, s="Trap ON/OFF X or Y Amp?", f=w1305) -> (s? t:f=w1298:i16)
        n976 = And(x="All FB On/Off", y="Feedback On/Off") -> (x .and. y?=w1296:cluster{"Set 1":bool, "Set 2":bool})
        n977 = local read "BD 1 Amplitude 1 (%)"() -> (w1316:dbl)
        n978 = local read "BD 1 Amplitude 2 (%)"() -> (w1315:dbl)
        n979 = local read "BD 1 Amplitude 3 (%)"() -> (w1314:dbl)
        n980 = Unbundle By Name(w1296) -> ("Set 1"=w1291:bool, "Set 2"=w1288:bool)
        n981 = local read "Y RF Amplitude Limits (%)"() -> (w1284:T16)
        n982 = local read "X RF Amplitude Limits (%)"() -> (w1285:T16)
        n983 = local read "BD 2 Amplitude 1 (%)"() -> (w1317:dbl)
        n984 = local read "BD 2 Amplitude 2 (%)"() -> (w1318:dbl)
        n985 = local read "BD 2 Amplitude 3 (%)"() -> (w1319:dbl)
        n986 = And(x="Trap 2 ON", y=w1288) -> (x .and. y?=w1286:bool)
        n987 = And(x="Trap 1 ON", y=w1291) -> (x .and. y?=w1289:bool)
        n988 = Multiply(x=w1303, y=w1316) -> (x*y=w1311:dbl)
        n989 = Multiply(x=w1315, y=w1302) -> (x*y=w1309:dbl)
        n990 = Multiply(x=w1314, y=w1301) -> (x*y=w1310:dbl)
        n991 = Multiply(x=w1317, y=w1300) -> (x*y=w1320:dbl)
        n992 = Multiply(x=w1318, y=w1299) -> (x*y=w1321:dbl)
        n993 = Multiply(x=w1319, y=w1298) -> (x*y=w1322:dbl)
        n994 = call "set RF board amplitude - interlace.vi"("Board 2 Amplitude Limits"=w1284, "Board 1 Amplitude Limits"=w1285, "error in"=w1312, "FPGA VI Reference In"=w1313, "Board 2 Amplitude 3 (%)"=w1322, "Board 1 Amplitude 3 (%)"=w1310, "Board 2 Amplitude 2 (%)"=w1321, "Board 2 Amplitude 1 (%)"=w1320, "Board 1 Amplitude 2 (%)"=w1309, "Board 1 Amplitude 1 (%)"=w1311) -> ("error out"=w1293:errorcluster, "FPGA VI Reference Out"=w1294:T19)
        n995 = xnode "Read/Write Control"("FPGA VI Reference In"=w1294, "error in"=w1293, "FB On/Off Set 1"=w1289, "FB On/Off Set 2"=w1286) -> ("error out"=w1292:errorcluster)  [unwired: 1 out]
      }
      event "Load parameters": Value Change {
        n996 = event-data() -> ()  [unwired: 7 out]
        n997 = property on="Saved AOD Raster Scan Parameter Sets" class="Arr (strict)"() -> ("Index Values"=w1333:u32[])  [unwired: 2 in, 2 out]
        n998 = Index Array(array=w1333, index=0) -> (element=w1330:u32)
        n999 = local write "Load parameters"(FALSE ("Load parameters")) -> ()
        n1000 = Index Array(array="Saved AOD Raster Scan Parameter Sets", index=w1330) -> (element=w1329:T26)
        n1001 = Unbundle By Name(w1329) -> ("Scan Range AOD (nm) 2"=w1328:dbl, "Step Size AOD (nm) 2"=w1327:dbl, "Scan Speed AOD (nm/s) 2"=w1326:dbl, "Number of scans (AOD) 2"=w1325:u16)
        n1002 = flat-sequence {
          tunnel: w1328 -> [w1336]
          tunnel: w1327 -> [w1335]
          tunnel: w1326 -> [w1334]
          tunnel: w1325 -> [w1337]
          frame #0 {
            n1003 = local write "Scan Speed (nm/s)"(w1334) -> ()
            n1004 = local write "Scan Range (nm)"(w1336) -> ()
            n1005 = local write "Step Size (nm)"(w1335) -> ()
          }
          frame #1 {
            n1006 = property on="Number of F/B Scans (AOD)" class="DigNum (strict)"("Val(Sgnl)"=w1337) -> ()  [unwired: 2 in, 2 out]
          }
        }
      }
      event "Trap 1 (ON/OFF)", "Trap 2 (ON/OFF)": Value Change {
        n1007 = event-data() -> ()  [unwired: 7 out]
        n1008 = property on="Trap 2 ON" class="Bool (strict)"("Val(Sgnl)"="Trap 2 (ON/OFF)") -> ()  [unwired: 2 in, 2 out]
        n1009 = property on="Trap 1 ON" class="Bool (strict)"("Val(Sgnl)"="Trap 1 (ON/OFF)") -> ()  [unwired: 2 in, 2 out]
      }
      event "DIO count 1 (ticks)", "DIO count 2 (ticks)", "DIO count 3 (ticks)", "Interlace", "Number Interlace Sets", "Not-Interlacing Set": Value Change {
        n1010 = event-data() -> ()  [unwired: 7 out]
        n1011 = local read "DIO count 3 (ticks)"() -> (w1350:u32)
        n1012 = local read "DIO count 1 (ticks)"() -> (w1352:u32)
        n1013 = local read "DIO count 2 (ticks)"() -> (w1351:u32)
        n1014 = To Unsigned Byte Integer(number="Not-Interlacing Set") -> (unsigned 8bit integer=w1341:u8)
        n1015 = Add(x=w1341, y=u8 1) -> (x+y=w1345:u8)
        n1016 = xnode "Read/Write Control"("FPGA VI Reference In"=w1356, "error in"=w1354, "DIO count 1 (ticks)"=w1352, "DIO count 2 (ticks)"=w1351, "DIO count 3 (ticks)"=w1350, "Interlace ON/OFF"="Interlace", "Number Interlace Cycles"="Number Interlace Sets", "Interlace Off Parameters"=w1345) -> ("error out"=w1355:errorcluster)  [unwired: 1 out]
        n1017 = Build Array(w1352, w1351, w1350) -> (w1343:u32[])
        n1018 = Split 1D Array(array=w1343, index="Number Interlace Sets") -> (first subarray=w1353:u32[])  [unwired: 1 out]
        n1019 = Index Array(array=w1343, index=w1341) -> (element=w1342:u32)
        n1020 = Add Array Elements(numeric array=w1353) -> (sum=w1347:u32)
        n1021 = Select(t=w1347, s="Interlace", f=w1342) -> (s? t:f=→"Total Counts (ticks)":u32)
      }
      event "Reset Feedback": Value Change {
        n1022 = event-data() -> ()  [unwired: 7 out]
        n1023 = Unbundle By Name("Reset Feedback") -> ("Set 1"=w1360:bool, "Set 2"=w1359:bool)
        n1024 = xnode "Read/Write Control"("FPGA VI Reference In"=w1362, "error in"=w1357, "FB Reset Set 1"=w1360, "FB Reset Set 2"=w1359) -> ("error out"=w1358:errorcluster)  [unwired: 1 out]
      }
      event "PID Gains": Value Change {
        n1025 = event-data() -> ()  [unwired: 7 out]
        n1026 = Unbundle By Name("PID Gains") -> ("Set 1"=w1366:T14, "Set 2"=w1365:T14)
        n1027 = xnode "Read/Write Control"("FPGA VI Reference In"=w1367, "error in"=w1363, "FB Gains Set 1"=w1366, "FB Gains Set 2"=w1365) -> ("error out"=w1364:errorcluster)  [unwired: 1 out]
      }
      event "AI2 to Setpoint", "Setpoints (V)": Value Change {
        n1028 = event-data() -> ()  [unwired: 7 out]
        n1029 = xnode "Read/Write Control"("FPGA VI Reference In"=w1373, "error in"=w1369) -> ("FPGA VI Reference Out"=w1372:T19, "error out"=w1371:errorcluster, "AI2 Y Sum Set 1"=w1380:i16, "AI2 Y Sum Set 2"=w1379:i16)
        n1030 = Cluster To Array(cluster="AI2 to Setpoint") -> (array=w1383:bool[])
        n1031 = local read "AI2 (V)"() -> (w1381:cluster{"Set 1":dbl, "Set 2":dbl})
        n1032 = Or Array Elements(Boolean array=w1383) -> (logical OR=w1384:bool)
        n1033 = Bundle By Name(cluster=w1381, "Set 1"=w1380, "Set 2"=w1379) -> (w1378:cluster{"Set 1":dbl, "Set 2":dbl})
        n1034 = Divide(x=w1378, y=3276.7) -> (x/y=w1377:cluster{"Set 1":dbl, "Set 2":dbl})
        "AI2 (V)" <- w1377
        n1035 = case shown="True" w1384 {
          tunnel: [w1387 w1404] -> w1376
          tunnel: "AI2 to Setpoint" -> [_ w1400]
          tunnel: "Setpoints (V)" -> [w1388 w1403]
          tunnel: w1377 -> [_ w1397]
          frame False {
            n1036 = Multiply(x=3276.7, y=w1388) -> (x*y=w1389:cluster{"Set 1":dbl, "Set 2":dbl})
            n1037 = To Word Integer(number=w1389) -> (16bit integer=w1387:cluster{"Set 1":i16, "Set 2":i16})
          }
          frame True {
            n1038 = Unbundle By Name(w1397) -> ("Set 1"=w1396:dbl, "Set 2"=w1395:dbl)
            n1039 = Unbundle By Name(w1403) -> ("Set 1"=w1402:dbl, "Set 2"=w1401:dbl)
            n1040 = Unbundle By Name(w1400) -> ("Set 1"=w1399:bool, "Set 2"=w1398:bool)
            n1041 = Select(t=w1396, s=w1399, f=w1402) -> (s? t:f=w1394:dbl)
            n1042 = Select(t=w1395, s=w1398, f=w1401) -> (s? t:f=w1393:dbl)
            n1043 = Bundle By Name(cluster=w1403, "Set 1"=w1394, "Set 2"=w1393) -> (w1391:cluster{"Set 1":dbl, "Set 2":dbl})
            n1044 = local write "Setpoints (V)"(w1391) -> ()
            n1045 = Multiply(x=3276.7, y=w1391) -> (x*y=w1392:cluster{"Set 1":dbl, "Set 2":dbl})
            n1046 = To Word Integer(number=w1392) -> (16bit integer=w1404:cluster{"Set 1":i16, "Set 2":i16})
          }
        }
        n1047 = Unbundle By Name(w1376) -> ("Set 1"=w1375:i16, "Set 2"=w1374:i16)
        n1048 = xnode "Read/Write Control"("FPGA VI Reference In"=w1372, "error in"=w1371, "FB Setpoint Set 1"=w1375, "FB Setpoint Set 2"=w1374) -> ("error out"=w1370:errorcluster)  [unwired: 1 out]
      }
      event "Invert GI": Value Change {
        n1049 = event-data() -> ()  [unwired: 7 out]
        n1050 = xnode "Read/Write Control"("FPGA VI Reference In"=w1409, "error in"=w1407, "Invert GI"="Invert GI", "Invert GI 2"="Invert GI") -> ("error out"=w1408:errorcluster)  [unwired: 1 out]
      }
      event "Green FB Setpoint (mV)", "Green FB Gains", "Green FB On/Off", "Current When FB OFF (%)", "Green int current ON count adj": Value Change {
        n1051 = event-data() -> ()  [unwired: 7 out]
        n1052 = local read "Green FB Setpoint (mV)"() -> (w1416:dbl)
        n1053 = local read "Current When FB OFF (%)"() -> (w1419:dbl)
        n1054 = Multiply(x=w1416, y=3.2767) -> (x*y=w1415:dbl)
        n1055 = Multiply(x=w1419, y=655.35) -> (x*y=w1420:dbl)
        n1056 = To Unsigned Word Integer(number=w1420) -> (unsigned 16bit integer=w1418:u16)
        n1057 = local read "Green int current ON count adj"() -> (w1423:u32)
        n1058 = local read "Green FB Gains"() -> (w1422:T14)
        n1059 = local read "Green ON/Interlacing"() -> (w1413:bool)
        n1060 = local read "Green laser mode"() -> (w1412:enum32{"Laser ON", "Laser OFF", "Interlace"})
        n1061 = local read "Green FB On/Off"() -> (w1424:bool)
        n1062 = Equal?(x=w1412, y=enum32{"Laser ON", "Laser OFF", "Interlace"}."Interlace") -> (x = y?=w1410:bool)
        n1063 = Compound Arithmetic op=AND(w1410, w1424, w1413) -> (w1414:bool)
        n1064 = xnode "Read/Write Control"("FPGA VI Reference In"=w1427, "error in"=w1426, "Green FB Setpoint"=w1415, "Green FB On/Off"=w1414, "Current Out"=w1418, "Green int current ON count adj"=w1423, "Green FB Gains"=w1422) -> ("error out"=w1425:errorcluster)  [unwired: 1 out]
      }
      event "Green laser mode", "Green ON/Interlacing": Value Change {
        n1065 = event-data() -> ()  [unwired: 7 out]
        n1066 = local write "Green Laser ON/OFF"("Green ON/Interlacing") -> ()
        n1067 = case shown="True" "Green ON/Interlacing" {
          tunnel: "Green laser mode" -> [_ w1441]
          tunnel: [enum32{"Laser ON", "Laser OFF", "Interlace"}."Laser OFF" ("Green laser mode") w1441] -> w1430
          tunnel: [FALSE w1437] -> w1429
          frame False {
          }
          frame True {
            n1068 = local read "Green FB On/Off"() -> (w1438:bool)
            n1069 = Equal?(x=w1441, y=enum32{"Laser ON", "Laser OFF", "Interlace"}."Interlace") -> (x = y?=w1439:bool)
            n1070 = And(x=w1439, y=w1438) -> (x .and. y?=w1437:bool)
          }
        }
        n1071 = xnode "Read/Write Control"("FPGA VI Reference In"=w1434, "error in"=w1432, "Operating Mode"=w1430, "Operating Mode 2"=w1430, "Green FB On/Off"=w1429) -> ("error out"=w1433:errorcluster)  [unwired: 1 out]
      }
      event "Green Laser ON/OFF": Value Change {
        n1072 = event-data() -> ()  [unwired: 7 out]
        n1073 = property on="Green ON/Interlacing" class="Bool (strict)"("Val(Sgnl)"="Green Laser ON/OFF") -> ()  [unwired: 2 in, 2 out]
      }
      event "Test ttrig": Value Change {
        n1074 = event-data() -> ()  [unwired: 7 out]
        n1075 = xnode "Read/Write Control"("FPGA VI Reference In"=w1446, "error in"=w1445, "TTrig?"=TRUE) -> ("error out"=w1444:errorcluster)  [unwired: 1 out]
      }
      event "Neg. TTrig FPGA": Value Change {
        n1076 = event-data() -> ()  [unwired: 7 out]
        n1077 = xnode "Read/Write Control"("FPGA VI Reference In"=w1450, "error in"=w1449, "TTrig Negate Pos"="Neg. TTrig FPGA") -> ()  [unwired: 2 out]
      }
      event "- phase (APD 1 Gate)", "+ phase (APD 1 Gate)": Value Change {
        n1078 = event-data() -> ()  [unwired: 7 out]
        n1079 = local read "Phase Adj. (APD 1 Gate)"() -> (w1451:i16)
        n1080 = Negate(x=w1451) -> (-x=w1459:i16)
        n1081 = Select(t=w1459, s="- phase (APD 1 Gate)", f=w1451) -> (s? t:f=w1458:i16)
        n1082 = Or(x="- phase (APD 1 Gate)", y="+ phase (APD 1 Gate)") -> (x .or. y?=w1454:bool)
        n1083 = xnode "Read/Write Control"("FPGA VI Reference In"=w1461, "error in"=w1460, "Phase count adjustment (APD 1 Gate)"=w1458) -> ("FPGA VI Reference Out"=w1456:T19, "error out"=w1457:errorcluster)
        n1084 = xnode "Read/Write Control"("FPGA VI Reference In"=w1456, "error in"=w1457, "+ phase (APD 1 Gate)"=w1454) -> ("error out"=w1455:errorcluster)  [unwired: 1 out]
      }
      event "+ phase (APD 2 Gate)", "- phase (APD 2 Gate)": Value Change {
        n1085 = event-data() -> ()  [unwired: 7 out]
        n1086 = local read "Phase Adj. (APD 2 Gate)"() -> (w1462:i16)
        n1087 = Negate(x=w1462) -> (-x=w1470:i16)
        n1088 = Select(t=w1470, s="- phase (APD 2 Gate)", f=w1462) -> (s? t:f=w1469:i16)
        n1089 = Or(x="- phase (APD 2 Gate)", y="+ phase (APD 2 Gate)") -> (x .or. y?=w1465:bool)
        n1090 = xnode "Read/Write Control"("FPGA VI Reference In"=w1472, "error in"=w1471, "Phase count adjustment (APD 2 Gate)"=w1469) -> ("FPGA VI Reference Out"=w1467:T19, "error out"=w1468:errorcluster)
